vi "유턴 라바콘 좌표.vi"() -> ()   [LabVIEW 2016]
uses:
  <vilib>/Platform/TimedLoop/XDataNode/timing_clust.ctl
  <vilib>/Platform/TimedLoop/XDataNode/nitl_modes.ctl
  <vilib>/Platform/TimedLoop/XDataNode/wakeup.ctl
  <vilib>/imath/engines/lvmath2/RunTimeEngine/Managers/WorkSpace/UID Generator.vi
  <vilib>/imath/engines/lvmath2/RunTimeEngine/BuiltInFunctions/size/NIMS_I32Row=size(GM).vi
  <instcachedir>/0/NIMS_I32Row=size(GM)_10ACDCB9F1F84A7E9F42C91D87611FB5.lvgen/NIMS_I32Row=size(GM)_10ACDCB9F1F84A7E9F42C91D87611FB5_001.vi
  <vilib>/imath/engines/lvmath2/RunTimeEngine/RunTimeType/NIMS_RunTimeType_From StrictType (excl LVString).vi
  <instcachedir>/0/NIMS_RunTimeType_From StrictType (excl LVString)_BBF44FB49F834B71AF7A14CCEDF8BECD.lvgen/NIMS_RunTimeType_From StrictType (excl LVString)_BBF44FB49F834B71AF7A14CCEDF8BECD_000.vi
  <vilib>/imath/engines/lvmath2/RunTimeEngine/LocalVariableDefStatement/MC_LocalVariableDefStatement_Display.vi
  <vilib>/imath/engines/lvmath2/RunTimeEngine/IndexRead/NIMS M(S,S).vi
  <instcachedir>/0/NIMS M(S,S)_AC51E74150A542F7991B9634C66F3096.lvgen/NIMS M(S,S)_AC51E74150A542F7991B9634C66F3096_002.vi
  <vilib>/imathl/engines/lvmath/Functions/Error Handling/Create Error.vi
  <vilib>/imath/engines/lvmath2/RunTimeEngine/Managers/SymbolTable/Clear UID.vi
  <vilib>/imath/engines/lvmath2/RunTimeEngine/NodeEndStatement/NIMS_NodeEndStatement_Output.vi
  <instcachedir>/0/NIMS_NodeEndStatement_Output_53EC0D466D134D7ABD903AC30B43404B.lvgen/NIMS_NodeEndStatement_Output_53EC0D466D134D7ABD903AC30B43404B_011.vi
  <vilib>/imath/engines/lvmath2/RunTimeEngine/ErrorHandling/NIMS_Finalize Error.vi
  <vilib>/imath/engines/lvmath2/RunTimeEngine/IndexRead/NIMS V(S).vi
  <instcachedir>/0/NIMS V(S)_0488751826AF41519A22953C041130DC.lvgen/NIMS V(S)_0488751826AF41519A22953C041130DC_002.vi
  <instcachedir>/0/NIMS M(S,S)_AC51E74150A542F7991B9634C66F3096.lvgen/NIMS M(S,S)_AC51E74150A542F7991B9634C66F3096_000.vi
  <vilib>/imath/engines/lvmath2/RunTimeEngine/IndexRead/NIMS M(R2,S).vi
  <instcachedir>/0/NIMS M(R2,S)_56813DCFDD5A484292D2195AF15D2BF5.lvgen/NIMS M(R2,S)_56813DCFDD5A484292D2195AF15D2BF5_000.vi
  <vilib>/imath/engines/lvmath2/RunTimeEngine/ArithmeticOperatorToken/NIMS_ArithmeticOperator_minus.vi
  <instcachedir>/0/NIMS_ArithmeticOperator_minus_E3B65B1D26A44BB184AFDC5B3F458E3D.lvgen/NIMS_ArithmeticOperator_minus_E3B65B1D26A44BB184AFDC5B3F458E3D_003.vi
  <vilib>/imath/engines/lvmath2/RunTimeEngine/ErrorHandling/NIMS_Create Error From Enums.vi
  <vilib>/imath/engines/lvmath2/RunTimeEngine/ArithmeticOperatorToken/NIMS_ArithmeticOperator_plus.vi
  <instcachedir>/0/NIMS_ArithmeticOperator_plus_0120E0498A0F4B4B9BDCAC2554767A4E.lvgen/NIMS_ArithmeticOperator_plus_0120E0498A0F4B4B9BDCAC2554767A4E_004.vi
  <instcachedir>/0/NIMS_NodeEndStatement_Output_53EC0D466D134D7ABD903AC30B43404B.lvgen/NIMS_NodeEndStatement_Output_53EC0D466D134D7ABD903AC30B43404B_002.vi
  <instcachedir>/0/NIMS_NodeEndStatement_Output_53EC0D466D134D7ABD903AC30B43404B.lvgen/NIMS_NodeEndStatement_Output_53EC0D466D134D7ABD903AC30B43404B_001.vi
  <instcachedir>/0/NIMS_NodeEndStatement_Output_53EC0D466D134D7ABD903AC30B43404B.lvgen/NIMS_NodeEndStatement_Output_53EC0D466D134D7ABD903AC30B43404B_005.vi
  <instcachedir>/0/NIMS_NodeEndStatement_Output_53EC0D466D134D7ABD903AC30B43404B.lvgen/NIMS_NodeEndStatement_Output_53EC0D466D134D7ABD903AC30B43404B_009.vi
  <vilib>/Platform/TimedLoop/XDataNode/XDataNode.xnode
  <vilib>/Platform/TimedLoop/XDataNode/XDNodeRunTimeDep.lvlib
  <vilib>/imath/engines/lvmath2/RunTimeEngine/Managers/SymbolTable/NIMS_WorkSpace.lvlib
panel:
  out "에러 출력":errorcluster
  out "오브젝트화된 배열(x,y)":T1
  out "y":dbl
  out "x":dbl
  in  "유턴 오브젝트 거리":dbl format="%#_13g"
  out "distance":dbl[](array[numeric])
  out "1사분면 오브젝트 배열":dbl[][](array[numeric])
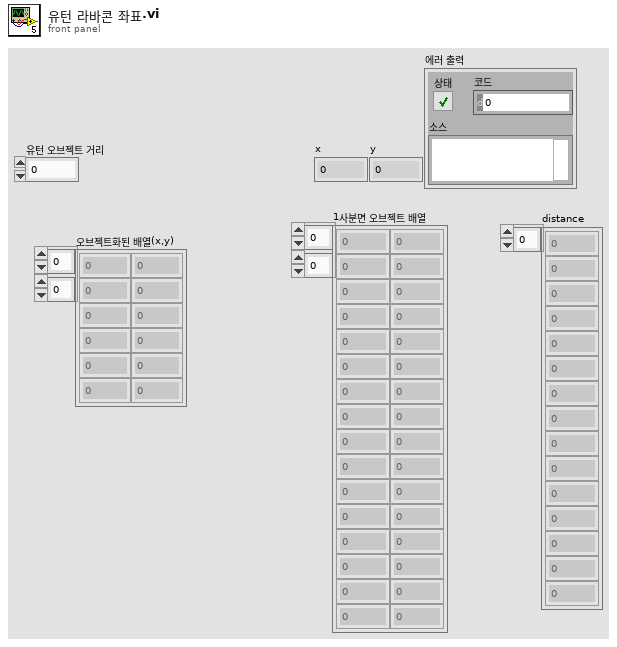
[diagram p1: front panel]
types:
  T1 = typedef "2차원배열 공유변수.ctl" = dbl[][]
  T2 = typedef "XDNodeRunTimeDep.lvlib/timing_clust.ctl" = cluster{"Expected End [f-1]":u64, "Actual End [f-1]":u64, "Finished Late? [f-1]":bool, "Expected End [i-1]":u64, "Actual End [i-1]":u64, "Finished Late? [i-1]":bool, "Expected Start [i]":u64, "Actual Start [i]":u64, "Expected Start [f]":u64, "Actual Start [f]":u64, "Source Name":string, "Structure Name":string, "Period":i64, "Deadline":i64, "Offset":i64, "Start":i64, "Priority":i32, "Timeout":i32, "Mode":T3, "Wakeup Reason":T4, "Error":errorcluster, "Source Type":string, "Secondary Source Type":string, "Global End Time":u64, "Global Start Time":u64, "Frame Duration":u64, "Iteration Duration":u64, "Assigned CPU":i32, "I/O Scan Engine Mode":u32}
  T3 = typedef "XDNodeRunTimeDep.lvlib/nitl_modes.ctl" = enum32{"No Change", "Process missed periods, maintain original phase", "Discard missed periods, maintain original phase", "Process missed periods, ignore original phase", "Discard missed periods, ignore original phase"}
  T4 = typedef "XDNodeRunTimeDep.lvlib/wakeup.ctl" = enum32{"Normal", "Aborted", "Asynchronous wakeup", "Timing source error", "Timed loop error", "Timeout"}
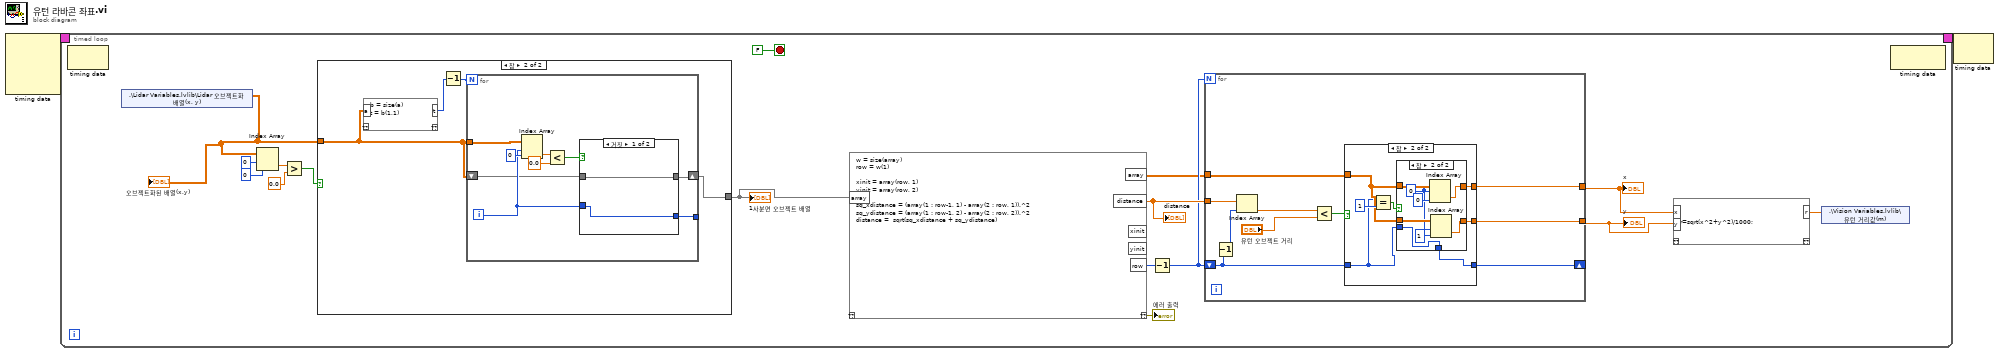
[diagram p0: block diagram]
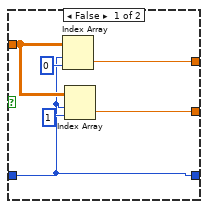
[diagram p2: hidden frame]
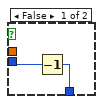
[diagram p3: hidden frame]
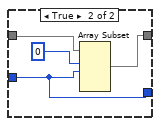
[diagram p5: hidden frame]
diagram:
  n1 = node-c288() -> (w2:T2)  [unwired: 4 in]
  n2 = timed-loop {
    timing: w2 -> [_]
    timing-out: [_] -> w1
    stop <- FALSE stop-if-true
    n3 = node-c288() -> ()  [unwired: 1 in, 1 out]
    n4 = shared-variable ".\\Lidar Variables.lvlib\\Lidar 오브젝트화 배열(x, y)"() -> (w4:T1)  [unwired: 1 in, 1 out]
    "오브젝트화된 배열(x,y)" <- w4
    n5 = Index Array(array=w4, index (row)=0 ("인덱스 (행)"), index (col)=0 ("비활성화된 인덱스 (열)")) -> (element=w16:dbl)
    n6 = Greater?(x=w16, y=0.0) -> (0:w14:bool)
    n7 = case shown="참" w14 {
      tunnel: w4 -> [w334 w336]
      tunnel: [w334 w337] -> w13
      frame False {
      }
      frame True {
        n8 = mathscript code="b = size(a)\nt = b(1,1)"("a"=w336) -> ("t"=w335:i32)  [unwired: 1 in, 1 out]
        n9 = Decrement(x=w335) -> (x-1=w338:i32)
        n10 = for {
          N: w338 -> [_]
          tunnel: w336 -> [w407]
          shift-right: [w404] -> w337
          shift-left: w336 -> [w405]
          tunnel: [w403] -> _
          i -> [w406]
          n11 = Index Array(array=w407, index (row)=w406, index (col)=0 ("비활성화된 인덱스 (열)")) -> (element=w410:dbl)
          n12 = Less?(x=w410, y=0.0) -> (x < y?=w408:bool)
          n13 = case shown="거짓" w408 {
            tunnel: w405 -> [w413 w417]
            tunnel: w406 -> [w412 w414]
            tunnel: [w413 w415] -> w404
            tunnel: [w412 w414] -> w403
            frame False {
            }
            frame True {
              n14 = Array Subset(array=w417, index (row)=0 ("인덱스"), length (row)=w414) -> (w415:T1)  [unwired: 2 in]
            }
          }
        }
      }
    }
    "1사분면 오브젝트 배열" <- w13
    n15 = mathscript code="w = size(array)\nrow = w(1)\n\nxinit = array(row, 1)\nyinit = array(row, 2)\n\nsq_xdistance = (array(1 : row-1, 1) - array(2 : row, 1)).^2\nsq_ydistance = (array(1 : row-1, 2) - array(2 : row, 2)).^2\ndistance =  sqrt(sq_xdistance + sq_ydistance)"("array"=w13) -> ("??"=→"에러 출력":errorcluster, "distance"=w11:dbl[], "row"=w10:i32, "array"=w8:dbl[][])  [unwired: 1 in, 2 out]
    "distance" <- w11
    n16 = Decrement(x=w10) -> (x-1=w9:i32)
    n17 = for {
      N: w9 -> [_]
      tunnel: w11 -> [w56]
      tunnel: w8 -> [w51]
      shift-right: [w47] -> _
      shift-left: w9 -> [w50]
      tunnel: [w49] -> w7
      tunnel: [w48] -> w6
      n18 = Decrement(x=w50) -> (x-1=w55:i32)
      n19 = Index Array(array=w56, index=w55) -> (element=w54:dbl)
      n20 = Less?(x=w54, y="유턴 오브젝트 거리") -> (x < y?=w52:bool)
      n21 = case shown="참" w52 {
        tunnel: w51 -> [w60 w67]
        tunnel: w50 -> [w57 w66]
        tunnel: [w59 w65] -> w49
        tunnel: [w58 w64] -> w48
        tunnel: [w57 w63] -> w47
        frame False {
          n22 = Index Array(array=w60, index (row)=w57, index (col)=0 ("비활성화된 인덱스 (열)")) -> (element=w59:dbl)
          n23 = Index Array(array=w60, index (row)=w57, index (col)=1 ("비활성화된 인덱스 (열)")) -> (element=w58:dbl)
        }
        frame True {
          n24 = Equal?(x=w66, y=1) -> (x = y?=w68:bool)
          n25 = case shown="참" w68 {
            tunnel: w67 -> [_ w77]
            tunnel: w67 -> [_ w76]
            tunnel: w66 -> [w71 w73]
            tunnel: [_ w75] -> w65
            tunnel: [_ w74] -> w64
            tunnel: [w70 w73] -> w63
            frame False {
              n26 = Decrement(x=w71) -> (x-1=w70:i32)
            }
            frame True {
              w72 = 0 ("비활성화된 인덱스 (행)")
              n27 = Index Array(array=w76, index (row)=w72, index (col)=0 ("비활성화된 인덱스 (열)")) -> (element=w75:dbl)
              n28 = Index Array(array=w77, index (row)=w72, index (col)=1 ("비활성화된 인덱스 (열)")) -> (element=w74:dbl)
            }
          }
        }
      }
    }
    "x" <- w7
    "y" <- w6
    n29 = mathscript code="r=sqrt(x^2+y^2)/1000;"("x"=w7, "y"=w6) -> ("r"=w5:cdb)  [unwired: 1 in, 1 out]
    n30 = shared-variable ".\\Vision Variables.lvlib\\유턴 거리값(m)"(w5) -> ()  [unwired: 1 in, 1 out]
    n31 = node-c288() -> ()  [unwired: 1 in, 1 out]
  }
  n32 = node-c288(w1) -> ()  [unwired: 1 out]
